vi "3-9.vi"   [LabVIEW 2022 SP3]
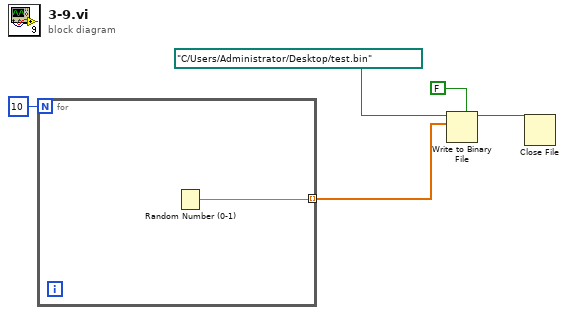
[diagram p0: block diagram]
diagram:
  n1 = for {
    N: 10 -> [_]
    tunnel: [w6] -> w1 mode=indexing
    n2 = Random Number (0-1)() -> (number: 0 to 1=w6:dbl)
  }
  n3 = Write to Binary File(file (use dialog)=path "C:/Users/Administrator/Desktop/test.bin" ("文件（使用对话框）"), data=w1, 5:FALSE ("预置数组或字符串大小？ (T)")) -> (refnum out=w2:refnum<file>)  [unwired: 3 in, 2 out]
  n4 = Close File(refnum=w2) -> ()  [unwired: 1 in, 2 out]
